vi "OAT Get CIC Filter Length.vi"(7 "CIC filter settings":T1(array[cluster])) -> (8 "filter length":i32[](array[numeric]))   [LabVIEW 2017, in "SoundVib_Resampling.lvlib"]
uses:
  <vilib>/addons/Sound and Vibration/Order Analysis/Resample Order Tracking/SoundVib_Resampling.lvlib
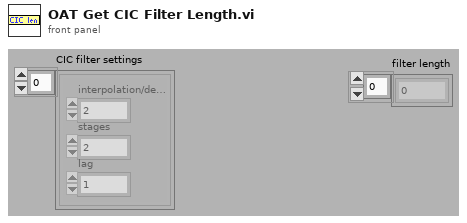
[diagram p1: front panel]
types:
  T1 = cluster{"interpolation/decimation factor":i32, "stages":i32, "lag":i32}[]
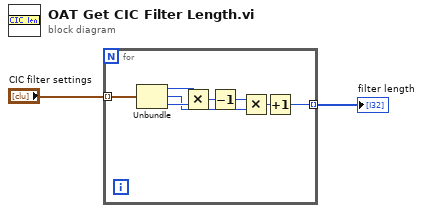
[diagram p0: block diagram]
diagram:
  n1 = for {
    tunnel: "CIC filter settings" -> [w10] mode=indexing
    tunnel: [w3] -> w1 mode=indexing
    n2 = Unbundle(w10) -> ("interpolation/decimation factor"=w6:i32, "stages"=w4:i32, "lag"=w5:i32)
    n3 = Multiply(x=w6, y=w5) -> (x*y=w9:i32)
    n4 = Decrement(x=w9) -> (x-1=w8:i32)
    n5 = Multiply(x=w8, y=w4) -> (x*y=w7:i32)
    n6 = Increment(x=w7) -> (x+1=w3:i32)
  }
  "filter length" <- w1
